vi "Temp Coef color converter.vi"(4 "Temp Coef":T1) -> (1 "Temp Coef to color":u32(colorbox))   [LabVIEW 2018, in "Enum to Color Converter.lvlib"]
uses:
  Temp Coef--control.ctl
  Enum to Color Converter.lvlib
  Resistor Band Colors/Resistor Band Colors.lvlib
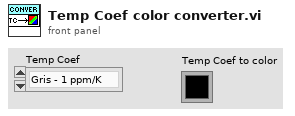
[diagram p1: front panel]
types:
  T1 = typedef "Temp Coef--control.ctl" = enum16{"Gris - 1 ppm/K", "Violeta - 5 ppm/K", "Azul - 10 ppm/K", "Verde - 20 ppm/K", "Amarillo - 25 ppm/K", "Naranja - 15 ppm/K", "Rojo - 50 ppm/K", "Marron - 100 ppm/K", "Negro - 250 ppm/K"}
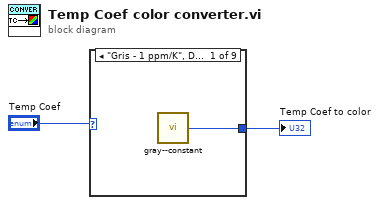
[diagram p0: block diagram]
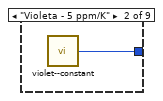
[diagram p2: hidden frame]
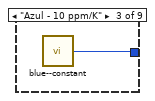
[diagram p3: hidden frame]
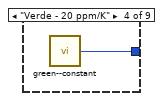
[diagram p4: hidden frame]
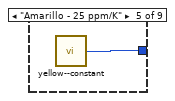
[diagram p5: hidden frame]
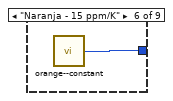
[diagram p6: hidden frame]
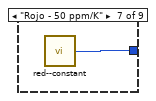
[diagram p7: hidden frame]
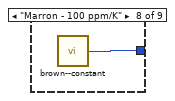
[diagram p8: hidden frame]
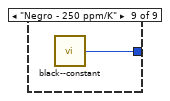
[diagram p9: hidden frame]
diagram:
  n1 = case shown="\"Gris - 1 ppm/K\", Default" "Temp Coef" {
    tunnel: [w3 w4 w5 w6 w7 w8 w9 w10 w11] -> w1
    frame "Gris - 1 ppm/K", Default {
      n2 = call "gray--constant.vi"() -> ("gray"=w3:u32)  [unwired: 5 in]
    }
    frame "Violeta - 5 ppm/K" {
      n3 = call "violet--constant.vi"() -> ("violet"=w4:u32)  [unwired: 5 in]
    }
    frame "Azul - 10 ppm/K" {
      n4 = call "blue--constant.vi"() -> ("blue"=w5:u32)  [unwired: 5 in]
    }
    frame "Verde - 20 ppm/K" {
      n5 = call "green--constant.vi"() -> ("green"=w6:u32)  [unwired: 5 in]
    }
    frame "Amarillo - 25 ppm/K" {
      n6 = call "yellow--constant.vi"() -> ("yellow"=w7:u32)  [unwired: 5 in]
    }
    frame "Naranja - 15 ppm/K" {
      n7 = call "orange--constant.vi"() -> ("orange"=w8:u32)  [unwired: 5 in]
    }
    frame "Rojo - 50 ppm/K" {
      n8 = call "red--constant.vi"() -> ("red"=w9:u32)  [unwired: 5 in]
    }
    frame "Marron - 100 ppm/K" {
      n9 = call "brown--constant.vi"() -> ("brown"=w10:u32)  [unwired: 5 in]
    }
    frame "Negro - 250 ppm/K" {
      n10 = call "black--constant.vi"() -> ("Negro"=w11:u32)  [unwired: 5 in]
    }
  }
  "Temp Coef to color" <- w1
